vi "Initialize Tag.vi"(6 "Units":string, 8 "error in (no error)":errorcluster, 9 "Data Type":string(combo), 10 "Tag Path":string, 11 "Logger in.lvclass":refnum<class "Logger.lvclass">) -> (0 "error out":errorcluster, 3 "Logger out.lvclass":refnum<class "Logger.lvclass">)   [LabVIEW 2017, in "Logger.lvclass"]
uses:
  Logger.lvclass
  Logger.lvclass/Logger.ctl
  <vilib>/Skyline/Tag/Wrapper/Wrapper_class/NI Skyline Tag.lvclass
  <vilib>/Skyline/Tag/Shared/typedefs/DataType.ctl
  <vilib>/Skyline/Tag/Wrapper/Wrapper AMQP_class/Open Tag AMQP.vi
  <vilib>/Skyline/Tag/Shared/NI Skyline Tag.lvlib
  <vilib>/Skyline/Tag/Wrapper/Wrapper AMQP_class/NI Skyline Tag AMQP.lvclass
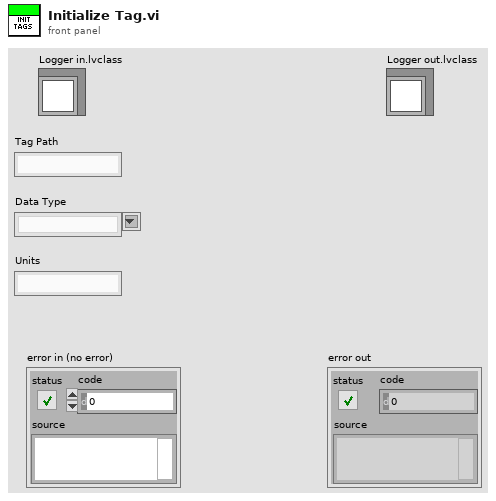
[diagram p1: front panel]
types:
  T1 = cluster{"Tag Units":string, "Tag Path":string, "Waveform":waveform(dbl), "Log":bool, "Tag Reference":refnum<class "NI Skyline Tag.lvclass">}
  T2 = typedef "NI Skyline Tag.lvlib/DataType.ctl" = enum32{"Double", "Integer", "String"}
  T3 = cluster{"Tag Units":string, "Tag Path":string, "Waveform":waveform(dbl), "Log":bool, "Tag Reference":refnum<class "NI Skyline Tag.lvclass">}[]
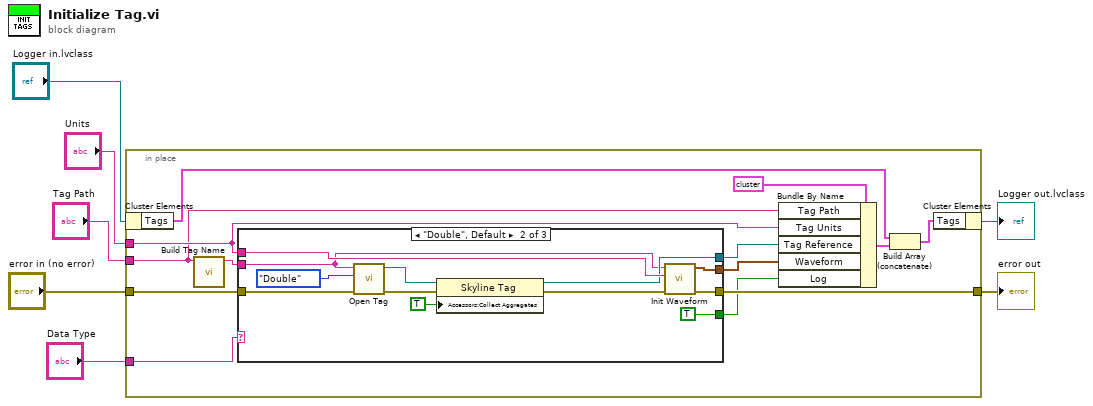
[diagram p0: block diagram]
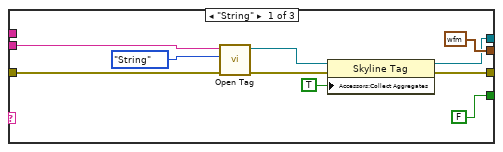
[diagram p2: hidden frame]
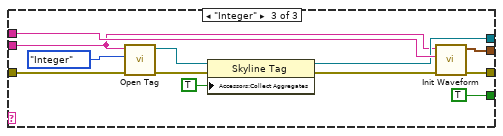
[diagram p3: hidden frame]
diagram:
  n1 = in-place {
    in-place-border: [w20] -> w7
    in-place-border: "Tag Path" -> [w10]
    in-place-border: "Data Type" -> [w19]
    in-place-border: "Units" -> [w17]
    in-place-border: "error in (no error)" -> [w9]
    n2 = in-place-cluster #1("Logger in.lvclass") -> ("Tags"=w13:T3)
    n3 = call "Build Tag Name.vi"("Tag"=w10) -> ("System Tag"=w14:string)  [unwired: 9 in, 1 out]
    n4 = case shown="\"Double\", Default" w19 {
      tunnel: w9 -> [w28 w35 w47]
      tunnel: [w21 w40 w52] -> w20
      tunnel: [w22 w32 w44] -> w18
      tunnel: [FALSE TRUE TRUE] -> w15
      tunnel: w17 -> [_ w38 w50]
      tunnel: [waveform(dbl) {"t0"=timestamp(0 s since 1904-01-01), "dt"=1.0, "Y"=[]} ("waveform") w39 w51] -> w16
      tunnel: w14 -> [w27 w31 w43]
      frame "String" {
        n5 = call-poly <vilib>:"Open Tag.vi"("error in (no error)"=w28, "data type"=DataType."String" ("Data Type"), "path"=w27) -> ("error out"=w23:errorcluster, "tag out"=w24:refnum<class "NI Skyline Tag.lvclass">)  [unwired: 7 in]
        n6 = property class="Skyline Tag"(reference=w24, error in=w23, "Accessors:Collect Aggregates"=TRUE ("Collect Aggregates")) -> (reference out=w22:refnum<class "NI Skyline Tag.lvclass">, error out=w21:errorcluster)
      }
      frame "Double", Default {
        n7 = call-poly <vilib>:"Open Tag.vi"("error in (no error)"=w35, "data type"=DataType."Double" ("Data Type"), "path"=w31) -> ("error out"=w34:errorcluster, "tag out"=w36:refnum<class "NI Skyline Tag.lvclass">)  [unwired: 7 in]
        n8 = property class="Skyline Tag"(reference=w36, error in=w34, "Accessors:Collect Aggregates"=TRUE ("Collect Aggregates")) -> (reference out=w32:refnum<class "NI Skyline Tag.lvclass">, error out=w33:errorcluster)
        n9 = call "Init Waveform.vi"("error in (no error)"=w33, "Units"=w38, "System Tag"=w31) -> ("error out"=w40:errorcluster, "waveform"=w39:waveform(dbl))  [unwired: 7 in]
      }
      frame "Integer" {
        n10 = call-poly <vilib>:"Open Tag.vi"("error in (no error)"=w47, "data type"=DataType."Integer" ("Data Type"), "path"=w43) -> ("error out"=w46:errorcluster, "tag out"=w48:refnum<class "NI Skyline Tag.lvclass">)  [unwired: 7 in]
        n11 = property class="Skyline Tag"(reference=w48, error in=w46, "Accessors:Collect Aggregates"=TRUE ("Collect Aggregates")) -> (reference out=w44:refnum<class "NI Skyline Tag.lvclass">, error out=w45:errorcluster)
        n12 = call "Init Waveform.vi"("error in (no error)"=w45, "Units"=w50, "System Tag"=w43) -> ("error out"=w52:errorcluster, "waveform"=w51:waveform(dbl))  [unwired: 7 in]
      }
    }
    n13 = Bundle By Name(cluster=T1 {"Tag Units"="", "Tag Path"="", "Waveform"={"t0"=timestamp(0 s since 1904-01-01), "dt"=1.0, "Y"=[]}, "Log"=FALSE, "Tag Reference"=refnum} ("Tag"), "Tag Path"=w10, "Tag Units"=w17, "Tag Reference"=w18, "Waveform"=w16, "Log"=w15) -> (w11:T1)
    n14 = Build Array (concatenate)(w13, w11) -> (w12:T3)
    n15 = in-place-cluster #1("Tags"=w12) -> (→"Logger out.lvclass":refnum<class "Logger.lvclass">)
  }
  "error out" <- w7
